vi "get Data Element.vi"(0 "LVx - Template Command in":refnum<class "REx - NART - Begin Point Calibration.lvclass">, 11 "error in (no error)":errorcluster) -> (4 "LVx - Template Command out":refnum<class "REx - NART - Begin Point Calibration.lvclass">, 6 "Calibrate Config":T1={"Frequency, MHz"=2412, "TX Gain"=62, "Data Rate"="1,0,0", "Packet Length"=1000, "Packet Count"=2000000}, 15 "error out":errorcluster)   [LabVIEW 2011, in "ART2 Test Panel.lvlib" / "REx - NART - Begin Point Calibration.lvclass"]
uses:
  REx - NART - Calibrate/REx - NART - Begin Point Calibration.lvclass
  Components/ART2.llb/NART/Controls/Calibrate Config.ctl
  Components/ART2.llb/CART/Controls/Data Rates.ctl
  REx - NART - Calibrate/REx - NART - Begin Point Calibration.lvclass/REx - NART - Begin Point Calibration.ctl
  ART2 Test Panel.lvlib
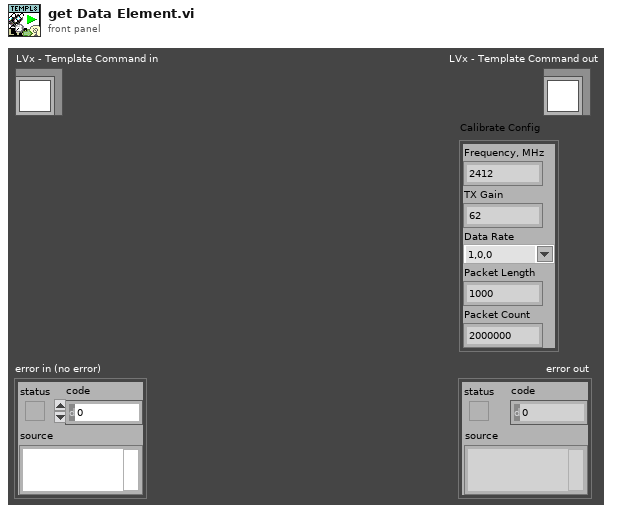
[diagram p1: front panel]
types:
  T1 = typedef "ART2 Test Panel.lvlib/Calibrate Config.ctl" = cluster{"Frequency, MHz":u32, "TX Gain":u32, "Data Rate":T2, "Packet Length":u32, "Packet Count":i32}
  T2 = typedef "ART2 Test Panel.lvlib/Data Rates.ctl" = string
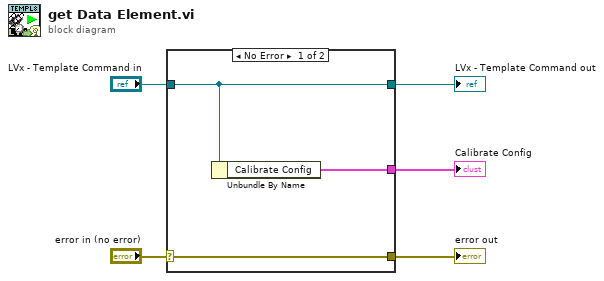
[diagram p0: block diagram]
diagram:
  n1 = case shown="No Error" "error in (no error)" {
    selector: "error in (no error)" -> [w8 w9]
    tunnel: [w8 w9] -> w4
    tunnel: [w6 w10] -> w2
    tunnel: "LVx - Template Command in" -> [w6 w10]
    tunnel: [w7 _] -> w1
    frame No Error {
      n2 = Unbundle By Name(w6) -> ("Calibrate Config"=w7:T1)
    }
    frame Error {
    }
  }
  "error out" <- w4
  "LVx - Template Command out" <- w2
  "Calibrate Config" <- w1
